vi "ExtractROI.vi"() -> ()   [LabVIEW 2016]
doc: "This example shows how to compute the histogram of an image or a region in the image. This example also shows how to set up and use the display tools to select and work on different regions in the image interactively."
uses:
  <vilib>/vision/NI_Vision_Development_Module.lvlib
panel:
  out "Image(ROI)":T1(plugin-control)
  out "Image":T1(plugin-control)
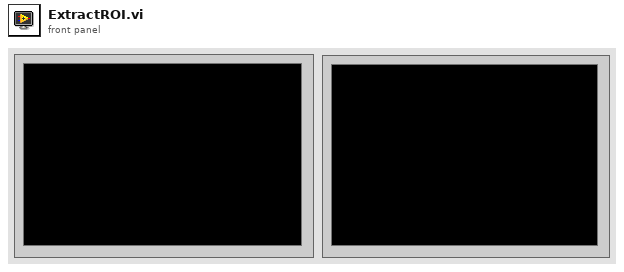
[diagram p1: front panel]
types:
  T1 = typedef "IMAQ Image.ctl" = refnum<image>
  T2 = typedef "IMAQ Rectangle" = cluster{"Left":i32, "Top":i32, "Right":i32, "Bottom":i32, "Rotation":dbl}
  T3 = typedef "ROI Descriptor" = cluster{"Global Rectangle":i32[], "Contours":cluster{"ID":enum32{"External", "Internal"}, "Type":u32, "Coordinates":i32[]}[]}
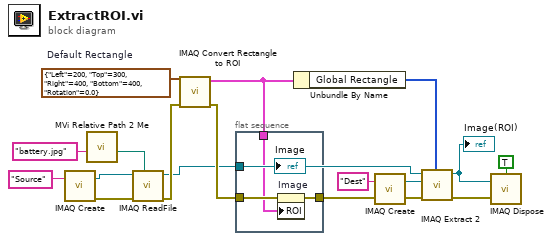
[diagram p0: block diagram]
diagram:
  w15 = T2 {"Left"=200, "Top"=300, "Right"=400, "Bottom"=400, "Rotation"=0.0}  # Default Rectangle
  n1 = call "IMAQ Create"("Image Name"="Source") -> ("New Image"=w18:T1, "error out"=w17:errorcluster)  [unwired: 4 in]
  n2 = call "MVi Relative Path 2 Me.vi"("Relative Path"="battery.jpg") -> ("Appended Dir"=w1:path)  [unwired: 5 in, 1 out]
  n3 = call "IMAQ ReadFile"("File Path"=w1, "error in (no error)"=w17, "Image"=w18) -> ("error out"=w14:errorcluster, "Image Out"=w5:T1)  [unwired: 4 in, 3 out]
  n4 = call "IMAQ Convert Rectangle to ROI"("error in (no error)"=w14, "Rectangle"=w15) -> ("error out"=w7:errorcluster, "ROI Descriptor"=w4:T3)  [unwired: 7 in]
  n5 = flat-sequence {
    tunnel: w7 -> [w22]
    tunnel: [w21] -> w6
    tunnel: w5 -> [w20]
    tunnel: w4 -> [w19]
    frame #0 {
      n6 = property on="Image" class="ImageControl"(error in=w22, "ROI"=w19) -> (error out=w21:errorcluster)  [unwired: 1 in, 1 out]
      "Image" <- w20
    }
  }
  n7 = Unbundle By Name(w4) -> ("Global Rectangle"=w13:i32[])
  n8 = call "IMAQ Create"("Image Name"="Dest", "error in (no error)"=w6) -> ("New Image"=w11:T1, "error out"=w8:errorcluster)  [unwired: 3 in]
  n9 = call "IMAQ Extract 2"("Optional Rectangle"=w13, "error in (no error)"=w8, "Image Dst"=w11, "Image Src"=w5) -> ("error out"=w10:errorcluster, "Image Dst Out"=w3:T1)  [unwired: 6 in]
  "Image(ROI)" <- w3
  n10 = call "IMAQ Dispose"("All Images? (No)"=TRUE, "Image"=w3, "error in (no error)"=w10) -> ()  [unwired: 3 in, 1 out]
